vi "Read Shared Variables.vi"(8 "error in (no error)":errorcluster caption="错误输入（无错误）", 11 "Message Queue":refnum<queue> caption="消息队列") -> (0 "Error Out":errorcluster caption="错误输出", 2 "Shared Variables":T1 caption="共享变量簇" {"System Time" format="%<%Y/%m/%d %H:%M:%S>T"}, 3 "dup Message Queue":refnum<queue> caption="消息队列副本")   [LabVIEW 2013]
uses:
  controls/Shared Variables.ctl
  support/Message Queue/Message Cluster.ctl
  Globals/Global - UI Stream and Variable Connections.vi
  support/Message Queue/Message Queue.lvlib
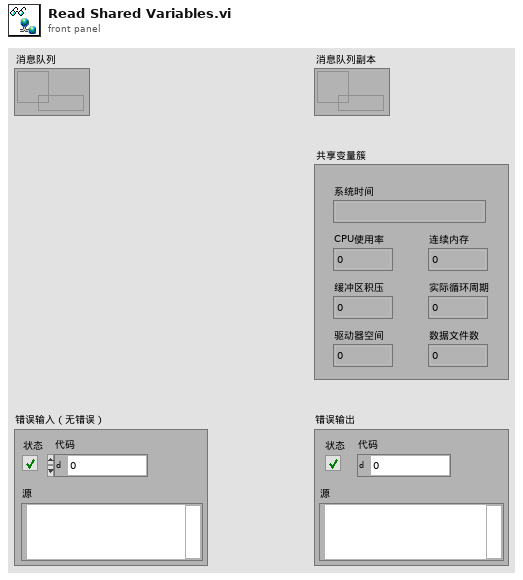
[diagram p1: front panel]
types:
  T1 = typedef "Shared Variables.ctl" = cluster{"System Time":timestamp, "CPU Usage":dbl, "Buffer Backlog":dbl, "Driver Space":dbl, "Contiguous Memory":dbl, "Actual Loop Period (ticks)":u32, "Number of Data Files":u32}
  T2 = typedef "Variable References.ctl" = cluster{"CPU Usage":refnum<k21>, "Contiguous Memory":refnum<k21>, "Actual Loop Period":refnum<k21>, "Buffer Backlog":refnum<k21>, "Drive Space":refnum<k21>, "Number of Data Files":refnum<k21>, "System Time":refnum<k21>}
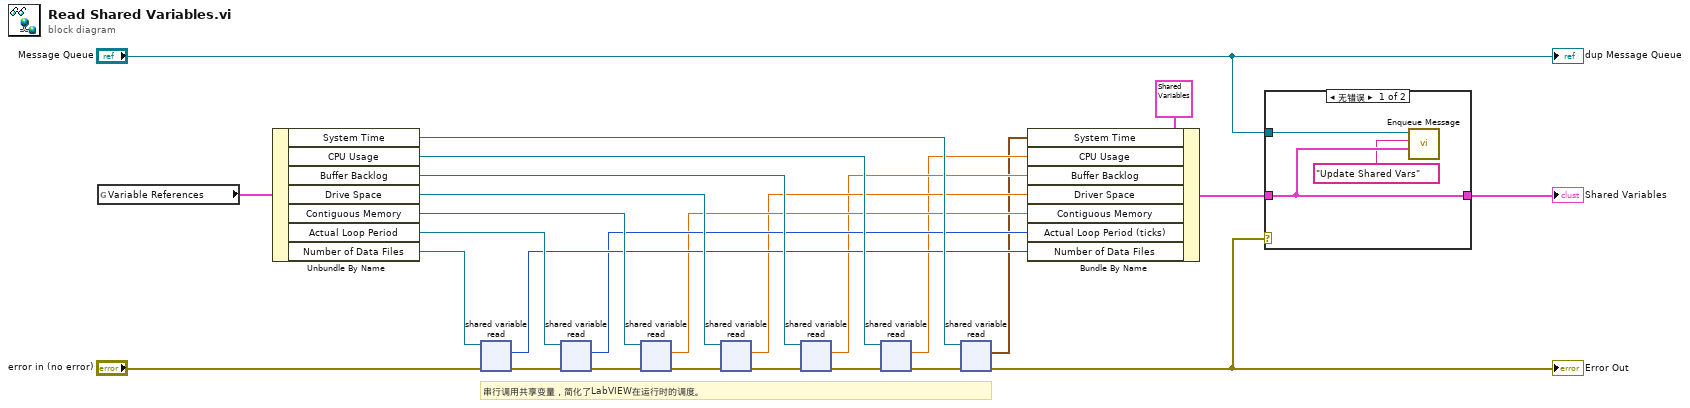
[diagram p0: block diagram]
diagram:
  # "串行调用共享变量，简化了LabVIEW在运行时的调度。"
  n1 = global read "Global - UI Stream and Variable Connections.vi" "Variable References"() -> (w21:T2)
  n2 = Unbundle By Name(w21) -> ("System Time"=w18:refnum<k21>, "CPU Usage"=w17:refnum<k21>, "Buffer Backlog"=w16:refnum<k21>, "Drive Space"=w15:refnum<k21>, "Contiguous Memory"=w14:refnum<k21>, "Actual Loop Period"=w13:refnum<k21>, "Number of Data Files"=w12:refnum<k21>)
  n3 = shared-variable-read(w12, "error in (no error)") -> (w22:errorcluster, w11:u32)  [unwired: 2 out]
  n4 = shared-variable-read(w13, w22) -> (w23:errorcluster, w10:u32)  [unwired: 2 out]
  n5 = shared-variable-read(w14, w23) -> (w24:errorcluster, w9:dbl)  [unwired: 2 out]
  n6 = shared-variable-read(w15, w24) -> (w25:errorcluster, w8:dbl)  [unwired: 2 out]
  n7 = shared-variable-read(w16, w25) -> (w26:errorcluster, w7:dbl)  [unwired: 2 out]
  n8 = shared-variable-read(w17, w26) -> (w27:errorcluster, w6:dbl)  [unwired: 2 out]
  n9 = shared-variable-read(w18, w27) -> (w4:errorcluster, w5:timestamp)  [unwired: 2 out]
  "Error Out" <- w4
  n10 = Bundle By Name(cluster=T1 {"System Time"=timestamp(0 s since 1904-01-01), "CPU Usage"=0.0, "Buffer Backlog"=0.0, "Driver Space"=0.0, "Contiguous Memory"=0.0, "Actual Loop Period (ticks)"=0, "Number of Data Files"=0} ("Shared Variables"), "System Time"=w5, "CPU Usage"=w6, "Buffer Backlog"=w7, "Driver Space"=w8, "Contiguous Memory"=w9, "Actual Loop Period (ticks)"=w10, "Number of Data Files"=w11) -> (w3:T1)
  n11 = case shown="无错误" w4 {
    tunnel: w3 -> [w29 w31]
    tunnel: "Message Queue" -> [w30 _]
    tunnel: [w29 w31] -> w1
    frame No Error {
      n12 = call "Enqueue Message.vi"("Message Data"=w29, "Message"="Update Shared Vars", "Message Queue"=w30) -> ()  [unwired: 7 in, 2 out]
    }
    frame Error {
    }
  }
  "Shared Variables" <- w1
  "dup Message Queue" <- "Message Queue"
